vi "json Insert Boolean - array path.vi"(8 "error in (no error)":errorcluster, 9 "anything":bool, 10 "path":string[](array[string]), 11 "JSON Document in":refnum<class "JSON Document.lvclass">) -> (0 "error out":errorcluster, 3 "JSON Document out":refnum<class "JSON Document.lvclass">)   [LabVIEW 2015, in "JSON Document.lvclass"]
uses:
  JSON Document.lvclass
  json Insert Boolean - string path.vi
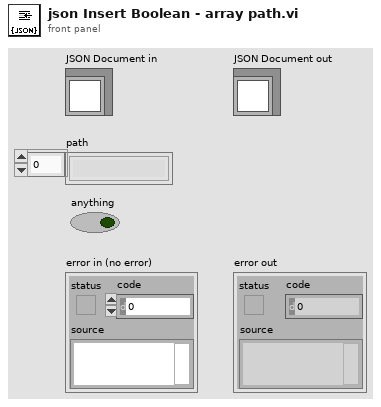
[diagram p1: front panel]
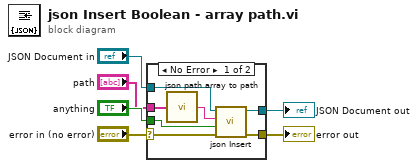
[diagram p0: block diagram]
diagram:
  n1 = case shown="No Error" "error in (no error)" {
    selector: "error in (no error)" -> [w8 w15]
    tunnel: [w7 w15] -> w5
    tunnel: [w12 w14] -> w3
    tunnel: "JSON Document in" -> [w11 w14]
    tunnel: "anything" -> [w9 _]
    tunnel: "path" -> [w13 _]
    frame No Error {
      n2 = call "json path array to path.vi"("path"=w13) -> ("String"=w10:string)
      n3 = call-poly "json Insert.vi"("error in (no error)"=w8, "anything"=w9, "path"=w10, "JSON Document in"=w11) -> ("error out"=w7:errorcluster, "JSON Document out"=w12:refnum<class "JSON Document.lvclass">)  [unwired: 6 in]
    }
    frame Error {
    }
  }
  "error out" <- w5
  "JSON Document out" <- w3
